vi "Acq_Reader.vi"(11 "AcqFileToRead":path) -> (1 "SamplingFreq":dbl, 2 "Data":ext[](array[numeric]), 3 "TimeLine":dbl[](array[numeric]))   [LabVIEW 2009]
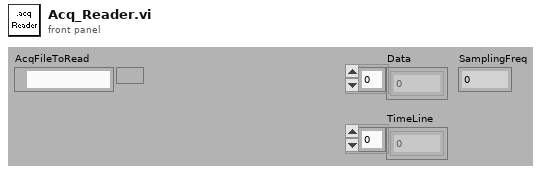
[diagram p1: front panel]
types:
  T1 = enum16{"big-endian, network order", "native, host order", "little-endian"}
  T2 = cluster{"WArr":dbl[], "VDiv":dbl, "VOff":dbl, "SRat":dbl}
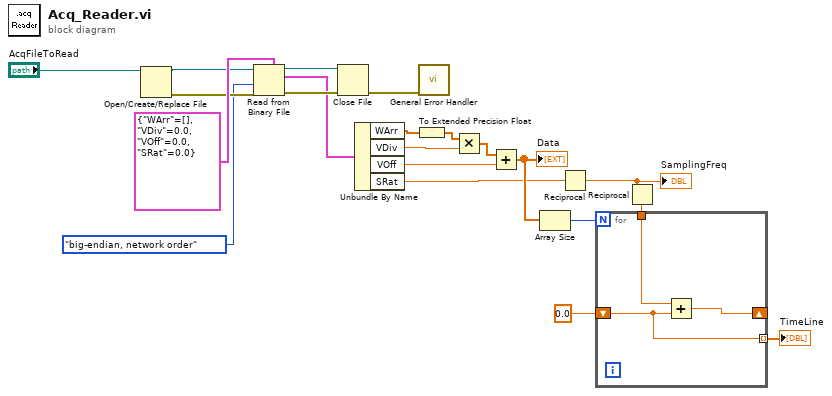
[diagram p0: block diagram]
diagram:
  n1 = Open/Create/Replace File(file path (use dialog)="AcqFileToRead") -> (refnum out=w17:refnum<file>, error out=w15:errorcluster)  [unwired: 5 in, 1 out]
  n2 = Read from Binary File(5:T2 {"WArr"=[], "VDiv"=0.0, "VOff"=0.0, "SRat"=0.0}, 8:w15, 9:T1."big-endian, network order" ("byte order (0:big-endian, network order)"), 11:w17) -> (0:w21:errorcluster, 2:w16:T2, 3:w20:refnum<file>)  [unwired: 2 in, 1 out]
  n3 = Close File(refnum=w20, error in=w21) -> (error out=w14:errorcluster)  [unwired: 1 out]
  n4 = Unbundle By Name(w16) -> ("WArr"=w13:dbl[], "VDiv"=w11:dbl, "VOff"=w10:dbl, "SRat"=w5:dbl)
  n5 = To Extended Precision Float(1:w13) -> (0:w12:ext[])
  n6 = call <vilib>:"General Error Handler.vi"("error in (no error)"=w14) -> ()  [unwired: 10 in, 5 out]
  n7 = Multiply(x=w12, y=w11) -> (x*y=w9:ext[])
  n8 = Add(x=w9, y=w10) -> (x+y=w7:ext[])
  "Data" <- w7
  n9 = Array Size(array=w7) -> (size(s)=w8:i32)
  n10 = Reciprocal(x=w5) -> (1/x=w4:dbl)
  "SamplingFreq" <- w4
  n11 = Reciprocal(x=w4) -> (1/x=w2:dbl)
  n12 = for {
    N: w8 -> [_]
    shift-right: [w24] -> _
    shift-left: 0.0 -> [w22]
    tunnel: w2 -> [w23]
    tunnel: [w22] -> w3 mode=indexing
    n13 = Add(x=w23, y=w22) -> (x+y=w24:dbl)
  }
  "TimeLine" <- w3
